vi "GetData.vi"(8 "error in (no error)":errorcluster, 11 "ChildSink in":refnum<class "ChildSink.lvclass">) -> (0 "error out":errorcluster, 2 "Data":dbl, 3 "ChildSink out":refnum<class "ChildSink.lvclass">)   [LabVIEW 2023, in "ChildSink.lvclass"]
uses:
  ChildSink.lvclass
  ChildSink.lvclass/ChildSink.ctl
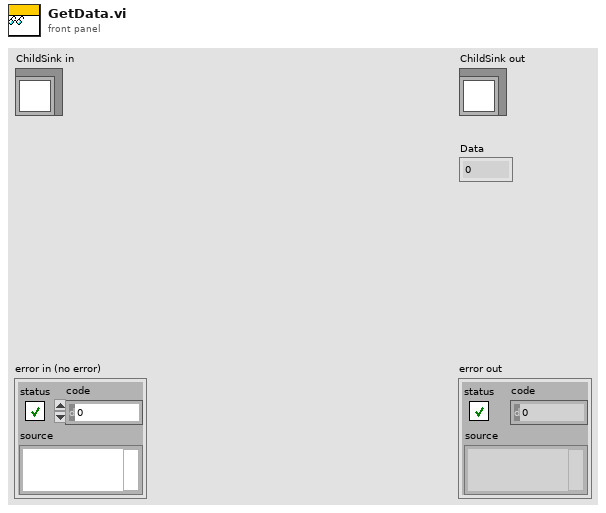
[diagram p1: front panel]
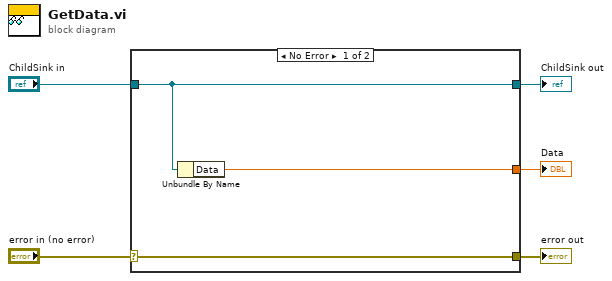
[diagram p0: block diagram]
diagram:
  n1 = case shown="No Error" "error in (no error)" {
    selector: "error in (no error)" -> [w8 w9]
    tunnel: [w8 w9] -> w4
    tunnel: [w7 w10] -> w2
    tunnel: "ChildSink in" -> [w7 w10]
    tunnel: [w6 _] -> w1
    frame No Error {
      n2 = Unbundle By Name(w7) -> ("Data"=w6:dbl)
    }
    frame Error {
    }
  }
  "error out" <- w4
  "ChildSink out" <- w2
  "Data" <- w1
